vi "Stop Message.vi"(8 "error in (no error)":errorcluster, 11 "LC Parser in":refnum<class "LC Parser.lvclass">) -> (0 "error out":errorcluster, 2 "Stop Message":T1, 3 "LC Parser out":refnum<class "LC Parser.lvclass">)   [LabVIEW 2020, in "RxnRover.lvlib" / "LC Parser.lvclass"]
uses:
  LC Parser.lvclass
  <userlib>/RxnRover/DynamicReentrant/src/Type Defs/Message.ctl
  Controller/Generic Plugin.lvclass
  LC Parser.lvclass/LC Parser.ctl
  <userlib>/RxnRover/DynamicReentrant/Dynamic Reentrant.lvlib
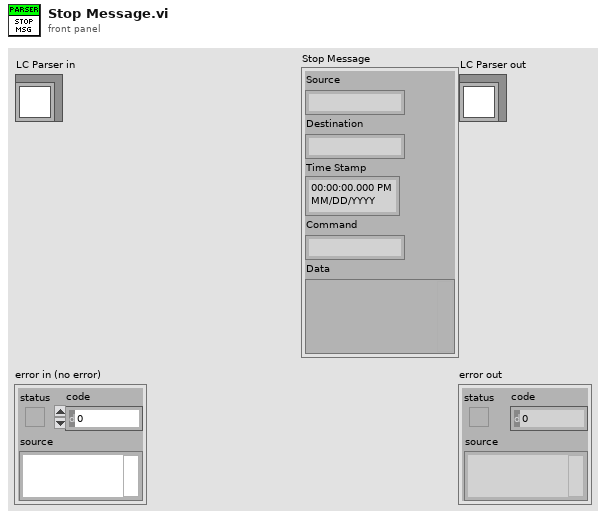
[diagram p1: front panel]
types:
  T1 = typedef "Dynamic Reentrant.lvlib/Message.ctl" = cluster{"Source":string, "Destination":string, "Time Stamp":timestamp, "Command":string, "Data":variant}
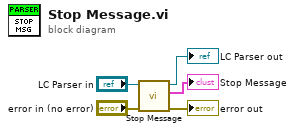
[diagram p0: block diagram]
diagram:
  n1 = call-parent "Stop Message.vi"("error in (no error)"="error in (no error)", "Generic Controller in"="LC Parser in") -> ("error out"=→"error out":errorcluster, "Stop Message"=→"Stop Message":T1, "Generic Controller out"=→"LC Parser out":refnum<class "LC Parser.lvclass">)  [unwired: 7 in]
